vi "Get Server State UE.vi"(11 "Template Server in":refnum<class "ctet_dmm.lvclass">) -> (2 "Server Internal State UE":refnum<user-event>, 3 "Template Server out":refnum<class "ctet_dmm.lvclass">)   [LabVIEW 2019, in "ctet_dmm.lvlib" / "ctet_dmm.lvclass"]
uses:
  ctet_dmm.lvclass
  typeDefs/Server State Data.ctl
  ctet_dmm.lvclass/ctet_dmm.ctl
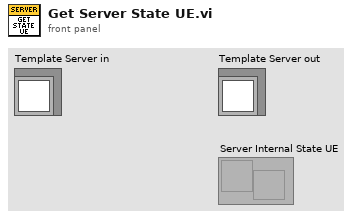
[diagram p1: front panel]
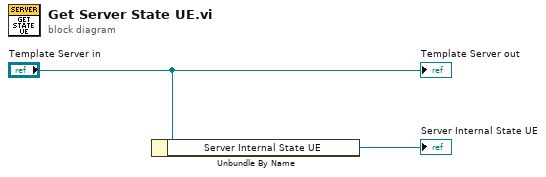
[diagram p0: block diagram]
diagram:
  n1 = Unbundle By Name("Template Server in") -> ("Server Internal State UE"=→"Server Internal State UE":refnum<user-event>)
  "Template Server out" <- "Template Server in"
